vi "Connect.vi"(8 "error in (no error)":errorcluster, 10 "Connection list in":string, 11 "Mock NI-SWITCH Consumer in":refnum<class "Mock %DEVICE% Consumer.lvclass">=refnum) -> (0 "error out":errorcluster, 3 "Mock NI-SWITCH Consumer out":refnum<class "Mock %DEVICE% Consumer.lvclass">)   [LabVIEW 2017, in "Mock %DEVICE% Consumer.lvclass"]
uses:
  Mock %DEVICE% Consumer.lvclass
  Mock %DEVICE% Consumer.lvclass/Mock %DEVICE% Consumer.ctl
  NI-SWITCH Consumer/NI-SWITCH Consumer.lvclass
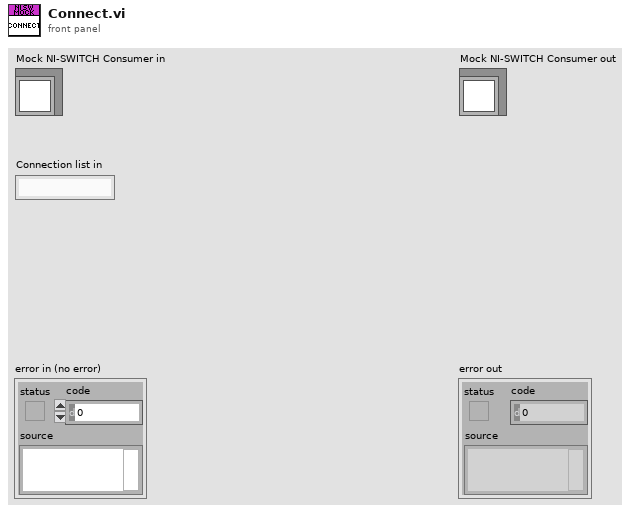
[diagram p1: front panel]
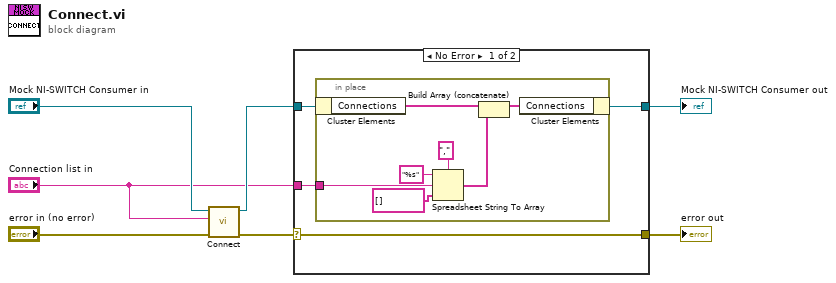
[diagram p0: block diagram]
diagram:
  n1 = call-parent "Connect.vi"("error in (no error)"="error in (no error)", "Connection list in"="Connection list in", "NI-SWITCH Consumer in"="Mock NI-SWITCH Consumer in") -> ("error out"=w4:errorcluster, "NI-SWITCH Consumer out"=w5:refnum<class "Mock %DEVICE% Consumer.lvclass">)  [unwired: 7 in]
  n2 = case shown="No Error" w4 {
    selector: w4 -> [w10 w20]
    tunnel: w5 -> [w11 w19]
    tunnel: [w10 w20] -> w3
    tunnel: [w9 w19] -> w2
    tunnel: "Connection list in" -> [w8 _]
    frame No Error {
      n3 = in-place {
        in-place-border: w8 -> [w16]
        n4 = in-place-cluster #1(w11) -> ("Connections"=w17:string[])
        n5 = Spreadsheet String To Array(delimiter (Tab)=",", format string="%s", spreadsheet string=w16, array type (2D Dbl)=string[] []) -> (array=w13:string[])
        n6 = Build Array (concatenate)(w17, w13) -> (w12:string[])
        n7 = in-place-cluster #1("Connections"=w12) -> (w9:refnum<class "Mock %DEVICE% Consumer.lvclass">)
      }
    }
    frame Error {
    }
  }
  "error out" <- w3
  "Mock NI-SWITCH Consumer out" <- w2
